vi "Calculate Roll Maneuver Step.vi"(9 "Roll":T1, 11 "Time":u32) -> (1 "Angle":dbl, 2 "Y":dbl, 3 "X":dbl, 4 "Total Time":i32)   [LabVIEW 2013]
uses:
  Dashboard UDP/Roll Maneuver.ctl
panel:
  out "Pct Complete":dbl
  out "Step":i16
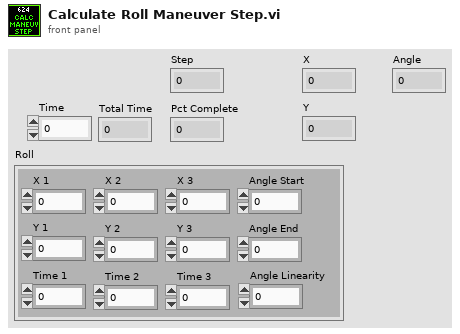
[diagram p1: front panel]
types:
  T1 = typedef "Roll Maneuver.ctl" = cluster{"X 1":dbl, "Y 1":dbl, "Y 2":dbl, "X 2":dbl, "Y 3":dbl, "X 3":dbl, "Time 1":i32, "Time 2":i32, "Time 3":i32, "Angle Start":dbl, "Angle End":dbl, "Angle Linearity":dbl}
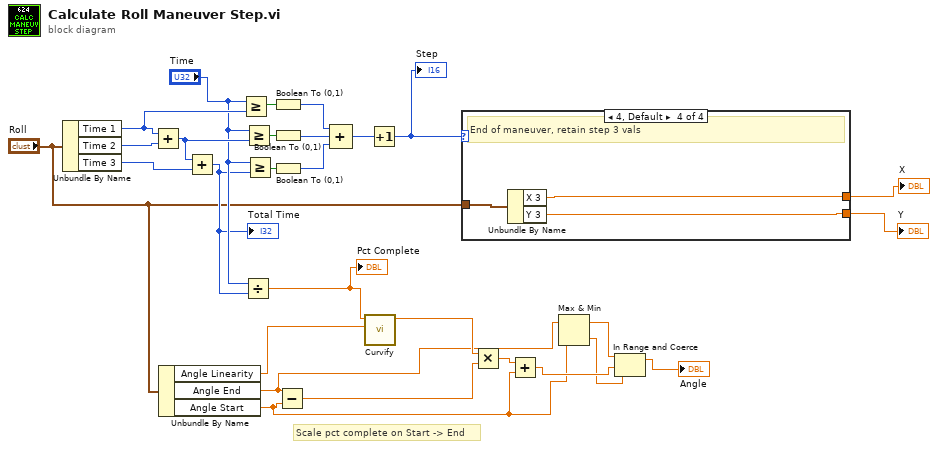
[diagram p0: block diagram]
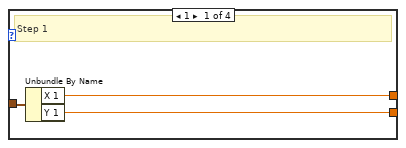
[diagram p2: hidden frame]
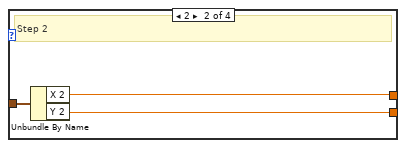
[diagram p3: hidden frame]
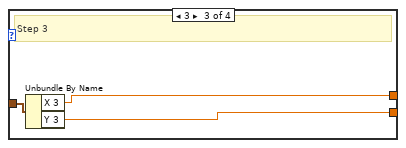
[diagram p4: hidden frame]
diagram:
  # "Scale pct complete on Start -> End"
  n1 = Unbundle By Name("Roll") -> ("Time 1"=w26:i32, "Time 2"=w28:i32, "Time 3"=w27:i32)
  n2 = Add(x=w26, y=w28) -> (x+y=w25:i32)
  n3 = Unbundle By Name("Roll") -> ("Angle Linearity"=w7:dbl, "Angle End"=w5:dbl, "Angle Start"=w4:dbl)
  n4 = Add(x=w25, y=w27) -> (x+y=w13:i32)
  "Total Time" <- w13
  n5 = Greater Or Equal?(x="Time", y=w26) -> (x >= y?=w24:bool)
  n6 = Divide(x="Time", y=w13) -> (x/y=w8:dbl)
  "Pct Complete" <- w8
  n7 = Greater Or Equal?(x="Time", y=w25) -> (x >= y?=w23:bool)
  n8 = Greater Or Equal?(x="Time", y=w13) -> (x >= y?=w22:bool)
  n9 = Boolean To (0,1)(Boolean=w24) -> (0, 1=w21:i16)
  n10 = Boolean To (0,1)(Boolean=w23) -> (0, 1=w20:i16)
  n11 = Boolean To (0,1)(Boolean=w22) -> (0, 1=w19:i16)
  n12 = Subtract(x=w5, y=w4) -> (x-y=w11:dbl)
  n13 = Compound Arithmetic op=ADD(w21, w20, w19) -> (w18:i16)
  n14 = call "Curvify.vi"("Linearity"=w7, "Numeric in"=w8) -> ("Numeric out"=w6:dbl)  [unwired: 9 in]
  n15 = Increment(x=w18) -> (x+1=w17:i16)
  "Step" <- w17
  n16 = case shown="4, Default" w17 {
    tunnel: "Roll" -> [w31 w34 w37 w40]
    tunnel: [w30 w33 w36 w39] -> w16
    tunnel: [w29 w32 w35 w38] -> w15
    frame 1 {
      # "Step 1"
      n17 = Unbundle By Name(w31) -> ("X 1"=w30:dbl, "Y 1"=w29:dbl)
    }
    frame 2 {
      # "Step 2"
      n18 = Unbundle By Name(w34) -> ("X 2"=w33:dbl, "Y 2"=w32:dbl)
    }
    frame 3 {
      # "Step 3"
      n19 = Unbundle By Name(w37) -> ("X 3"=w36:dbl, "Y 3"=w35:dbl)
    }
    frame 4, Default {
      # "End of maneuver, retain step 3 vals"
      n20 = Unbundle By Name(w40) -> ("X 3"=w39:dbl, "Y 3"=w38:dbl)
    }
  }
  "X" <- w16
  "Y" <- w15
  n21 = Multiply(x=w6, y=w11) -> (x*y=w10:dbl)
  n22 = Add(x=w10, y=w4) -> (x+y=w9:dbl)
  n23 = Max & Min(x=w5, y=w4) -> (max(x,y)=w3:dbl, min(x,y)=w2:dbl)
  n24 = In Range and Coerce(upper limit=w3, x=w9, lower limit=w2) -> (coerced(x)=→"Angle":dbl)  [unwired: 1 out]
